vi "Set String Buffer.vi"(10 "String Buffer":refnum<class "Buffer.lvclass">, 11 "Buffers in":refnum<class "Buffers.lvclass">) -> (3 "Buffers out":refnum<class "Buffers.lvclass">)   [LabVIEW 2017, in "DSF Core.lvlib" / "Buffers.lvclass"]
uses:
  Buffers.lvclass
  Buffer.lvclass
  Buffers.lvclass/Buffers.ctl
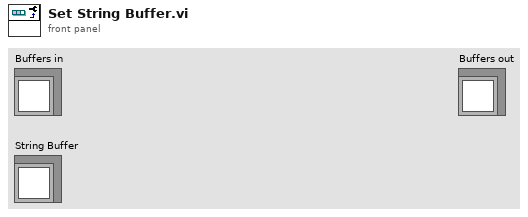
[diagram p1: front panel]
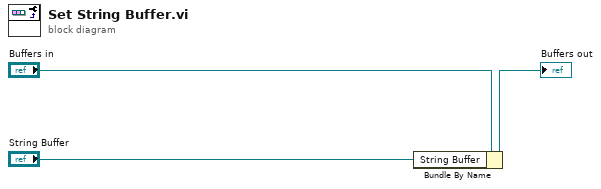
[diagram p0: block diagram]
diagram:
  n1 = Bundle By Name(cluster="Buffers in", "String Buffer"="String Buffer") -> (→"Buffers out":refnum<class "Buffers.lvclass">)
